vi "Initialize.vi"(8 "error in (no error)":errorcluster, 11 "VISA resource name":refnum<visa-resource-name>="COM1") -> (0 "error out":errorcluster, 3 "VISA resource name out":refnum<visa-resource-name>)   [LabVIEW 2012, in "Digikrom DK24x.lvlib"]
doc: "Initializes the serial port and returns a new VISA session."
uses:
  Digikrom DK24x.lvlib
  <vilib>/Instr/_visa.llb/VISA Configure Serial Port (Instr).vi
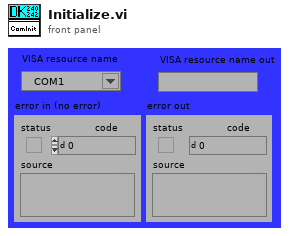
[diagram p1: front panel]
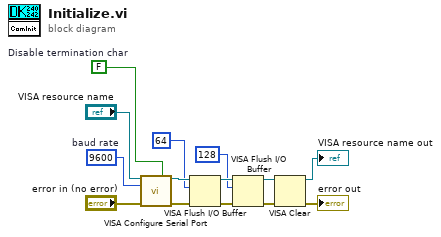
[diagram p0: block diagram]
diagram:
  w13 = u16 9600  # baud rate
  w6 = FALSE  # Disable termination char
  n1 = call-poly "VISA Configure Serial Port"("VISA resource name"="VISA resource name", "Enable Termination\nChar (T)"=w6, "baud rate (9600)"=w13, "error in (no error)"="error in (no error)") -> ("VISA resource name out"=w10:refnum<visa-resource-name>, "error out"=w11:errorcluster)  [unwired: 3 in, 7 out]
  n2 = VISA Flush I/O Buffer(VISA resource name=w10, mask (16)=64, error in (no error)=w11) -> (VISA resource name out=w9:refnum<visa-resource-name>, error out=w12:errorcluster)
  n3 = VISA Flush I/O Buffer(VISA resource name=w9, mask (16)=128, error in (no error)=w12) -> (VISA resource name out=w3:refnum<visa-resource-name>, error out=w4:errorcluster)
  n4 = VISA Clear(VISA resource name=w3, error in (no error)=w4) -> (VISA resource name out=→"VISA resource name out":refnum<visa-resource-name>, error out=→"error out":errorcluster)
